vi "Executable Get Version__icon_lib_labview_project_api.vi"(8 "error in (no error)":errorcluster, 11 "Build Spec Reference":refnum<vi>) -> (0 "error out":errorcluster, 2 "Version":T1, 3 "Build Spec Reference Dup":refnum<vi>)   [LabVIEW 2016, in "LabVIEW Project API__icon_lib_labview_project_api.lvlib"]
doc: "Returns a Build Specification Executable Version [Major, Minor, Fix, Build]\n\n<b>Author:</b> JG\n\n<b>ICON Technologies Pty Ltd</b>\nCopyright (C) 1990-2009\nAll Rights Reserved"
uses:
  LabVIEW Project API__icon_lib_labview_project_api.lvlib
panel:
  # "Output"
  # "Input"
  # "ICON Technologies Pty Ltd\nCopyright (C) 1990-2009\nAll Rights Reserved"
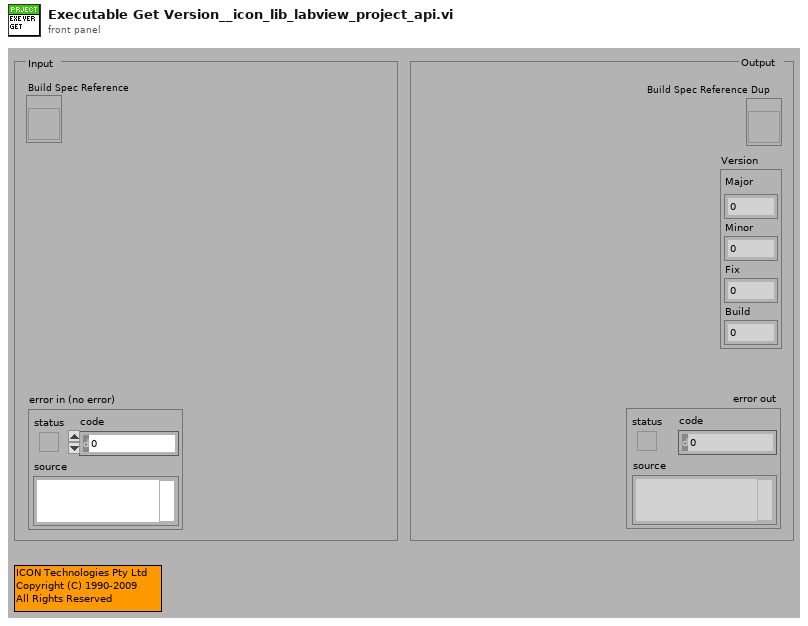
[diagram p1: front panel]
types:
  T1 = cluster{"Major":u16, "Minor":u16, "Fix":u16, "Build":u16}
  T2 = cluster{"[0]":u16, "[1]":u16, "[2]":u16, "[3]":u16}
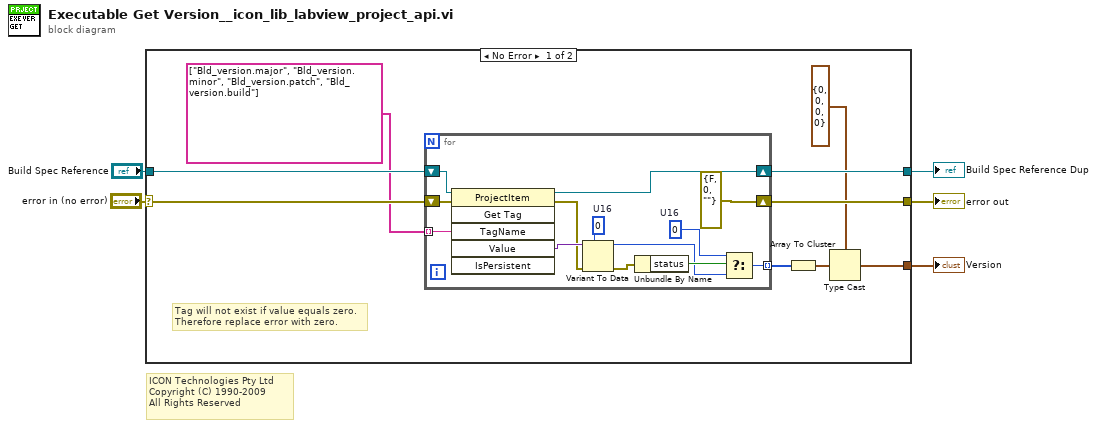
[diagram p0: block diagram]
diagram:
  # "ICON Technologies Pty Ltd\nCopyright (C) 1990-2009\nAll Rights Reserved"
  n1 = case shown="No Error" "error in (no error)" {
    selector: "error in (no error)" -> [w12 w29]
    tunnel: [w14 w29] -> w4
    tunnel: "Build Spec Reference" -> [w13 w28]
    tunnel: [w11 w28] -> w2
    tunnel: [w9 _] -> w1
    frame No Error {
      # "Tag will not exist if value equals zero.\nTherefore replace error with zero."
      n2 = for {
        shift-right: [w25] -> w11
        shift-left: w13 -> [w27]
        shift-right: [errorcluster {"status"=FALSE, "code"=0, "source"=""} ("error out")] -> w14
        shift-left: w12 -> [w26]
        tunnel: string[] ["Bld_version.major", "Bld_version.minor", "Bld_version.patch", "Bld_version.build"] -> [w24] mode=indexing
        tunnel: [w15] -> w8 mode=indexing
        w16 = u16 0  # U16
        w21 = u16 0  # U16
        n3 = invoke class="ProjectItem" method="Get Tag"(reference=w27, error in=w26, "TagName"=w24) -> (reference out=w25:refnum<vi>, error out=w22:errorcluster, "Value"=w23:variant)  [unwired: 3 in, 3 out]
        n4 = Variant To Data(error in=w22, type=w21, Variant=w23) -> (data=w17:u16, error out=w20:errorcluster)
        n5 = Unbundle By Name(w20) -> ("status"=w19:bool)
        n6 = Select(t=w16, s=w19, f=w17) -> (s? t:f=w15:u16)
      }
      n7 = Array To Cluster(array=w8) -> (cluster=w10:T2)
      n8 = Type Cast(type=T1 {"Major"=0, "Minor"=0, "Fix"=0, "Build"=0} ("Version 2"), x=w10) -> (*(type *) &x=w9:T1)
    }
    frame Error {
    }
  }
  "error out" <- w4
  "Build Spec Reference Dup" <- w2
  "Version" <- w1
